vi "Choreo_Util_AllianceFlipGetYearInfoNOT_DONE.vi"() -> (1 "FieldWidth_Meters":dbl=8.0692, 3 "FieldLength_Meters":dbl=16.541)   [LabVIEW 2019, in "ChoreoLib.lvlib"]
doc: "trajectory, mirrored across the field midline.\n\nInputs: \n - ChoreoTrajectory - cluster - Input trajectory\n\nOutputs:\n - Flipped Trajectory - cluster - trajectory, mirrored across the field midline."
uses:
  ChoreoLib.lvlib
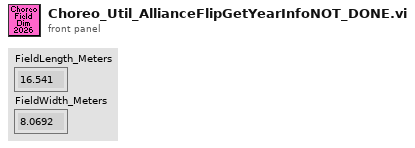
[diagram p1: front panel]
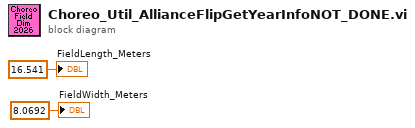
[diagram p0: block diagram]
diagram:
  "FieldLength_Meters" <- 16.541
  "FieldWidth_Meters" <- 8.0692
